vi "ReversedEngineering RemoveDirExtras.vi"(1 "Path":path) -> (15 "Path 2":path)   [LabVIEW 2016]
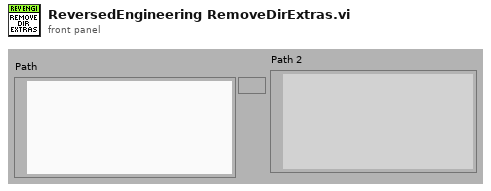
[diagram p1: front panel]
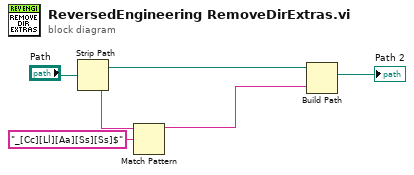
[diagram p0: block diagram]
diagram:
  n1 = Strip Path(path="Path") -> (stripped path=w1:path, name=w4:string)
  n2 = Match Pattern(string=w4, regular expression="_[Cc][Ll][Aa][Ss][Ss]$") -> (before substring=w2:string)  [unwired: 4 out]
  n3 = Build Path(base path=w1, name or relative path=w2) -> (appended path=→"Path 2":path)
